vi "set configuration by UID.vi"(8 "error in":errorcluster, 9 "configuration":refnum<class "CEF_serializable configuration.lvclass">, 10 "alias":string, 11 "CEF_HierarchyRepo in":refnum<class "CEF_HierarchyRepo.lvclass">) -> (0 "error out":errorcluster, 3 "CEF_HierarchyRepo out":refnum<class "CEF_HierarchyRepo.lvclass">)   [LabVIEW 2023, in "CEF.lvlib" / "CEF_HierarchyRepo.lvclass"]
doc: "Copyright 2017 National Instruments Corporation\n\nLicensed under the Apache License, Version 2.0 (the \"License\"); you may not use this file except in compliance with the License. You may obtain a copy of the License at http://www.apache.org/licenses/LICENSE-2.0\nUnless required by applicable law or agreed to in writing, software distributed under the License is distributed on an \"AS IS\" BASIS, WITHOUT WARRANTIES OR CONDITIONS OF ANY KIND, either express or implied. See the License for the specific language governing permissions and limitations under the License."
uses:
  CEF_HierarchyRepo.lvclass
  serializable configuration/CEF_serializable configuration.lvclass
  CEF_HierarchyRepo.lvclass/CEF_HierarchyRepo.ctl
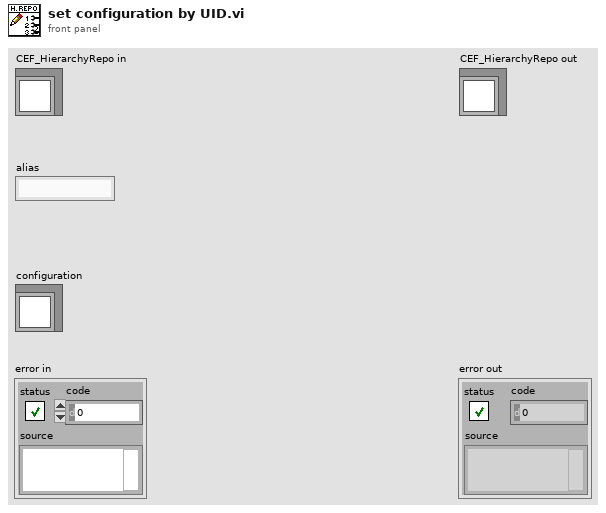
[diagram p1: front panel]
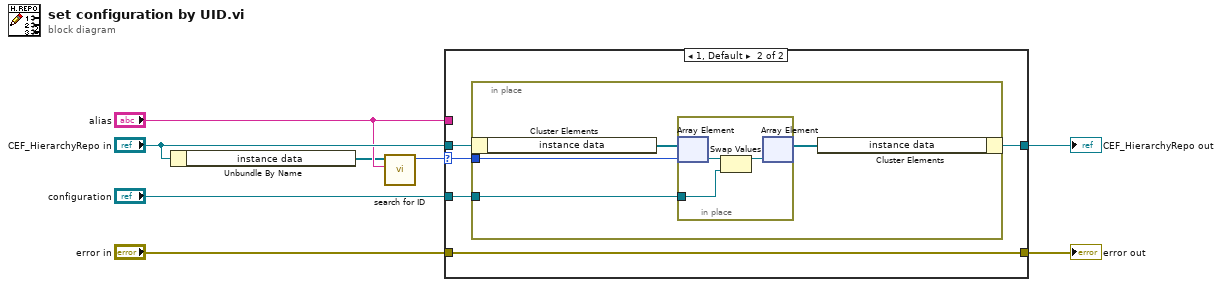
[diagram p0: block diagram]
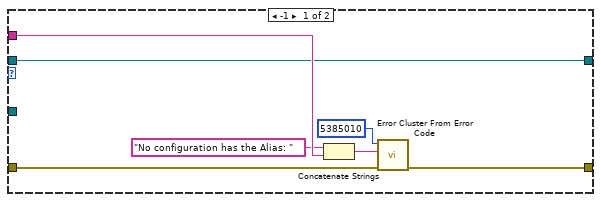
[diagram p2: hidden frame]
diagram:
  n1 = Unbundle By Name("CEF_HierarchyRepo in") -> ("instance data"=w1:refnum<class "CEF_serializable configuration.lvclass">[])
  n2 = call "search for ID.vi"("instance id"="alias", "instance data"=w1) -> ("index"=w2:i32)  [unwired: 9 in]
  n3 = case shown="1, Default" w2 {
    selector: w2 -> [_ w17]
    tunnel: "error in" -> [w15 w20]
    tunnel: [w14 w20] -> w7
    tunnel: "alias" -> [w11 _]
    tunnel: "configuration" -> [_ w16]
    tunnel: "CEF_HierarchyRepo in" -> [w9 w19]
    tunnel: [w9 w18] -> w5
    frame -1 {
      n4 = Concatenate Strings("No configuration has the Alias: " ("string"), w11) -> (w12:string)
      n5 = call <vilib>:"Error Cluster From Error Code.vi"("error in (no error)"=w15, "error message (\"\")"=w12, "error code (0)"=5385010) -> ("error out"=w14:errorcluster)  [unwired: 6 in]
    }
    frame 1, Default {
      n6 = in-place {
        in-place-border: w17 -> [w22]
        in-place-border: w16 -> [w21]
        n7 = in-place-cluster #1(w19) -> ("instance data"=w24:refnum<class "CEF_serializable configuration.lvclass">[])
        n8 = in-place {
          in-place-border: w21 -> [w26]
          n9 = in-place-array #2(w24, w22) -> (w27:refnum<class "CEF_serializable configuration.lvclass">)
          n10 = Swap Values(12:w27, 14:w26) -> (1:w25:refnum<class "CEF_serializable configuration.lvclass">)  [unwired: 1 in, 1 out]
          n11 = in-place-array #2(w25) -> (w23:refnum<class "CEF_serializable configuration.lvclass">[])  [unwired: 1 out]
        }
        n12 = in-place-cluster #1("instance data"=w23) -> (w18:refnum<class "CEF_HierarchyRepo.lvclass">)
      }
    }
  }
  "error out" <- w7
  "CEF_HierarchyRepo out" <- w5
